vi "T7MOD_Write_with_Readback_UINT16_Register.vi"(6 "Timeout":u32=1000, 7 "UINT16 to Write":u16, 8 "error in":errorcluster, 9 "LabJack UINT16 Register":i32=55110, 10 "Remote Port":u16=502, 11 "Remote IP Address":string="192.168.1.15") -> (0 "error out":errorcluster, 1 "Written At":timestamp, 3 "nIter":i32)   [LabVIEW 2016]
panel:
  # "Input"
  # "TCP Parameters"
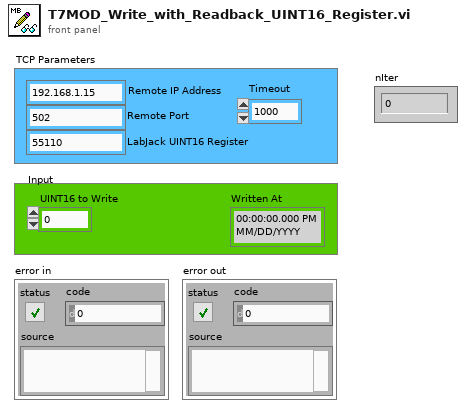
[diagram p1: front panel]
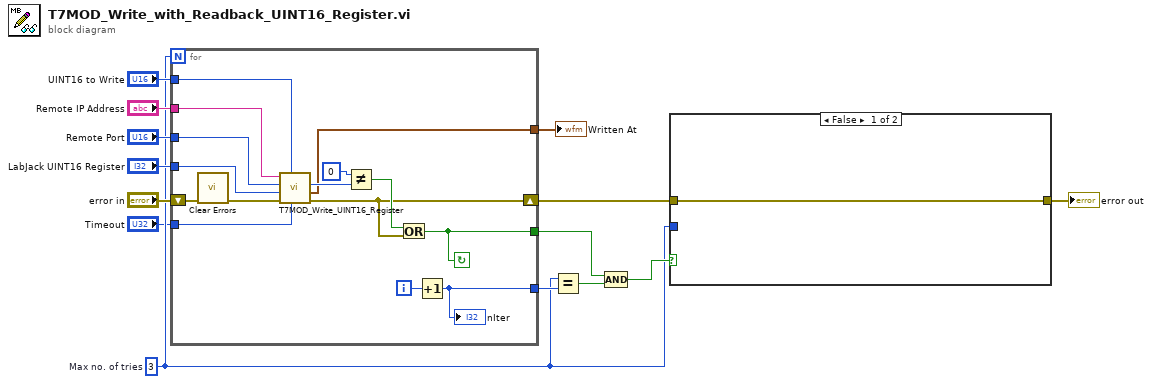
[diagram p0: block diagram]
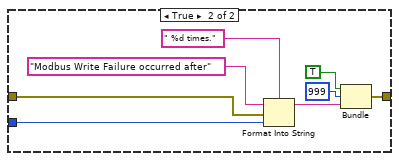
[diagram p2: hidden frame]
diagram:
  w6 = 3  # Max no. of tries
  n1 = for {
    N: w6 -> [_]
    tunnel: "Remote IP Address" -> [w29]
    shift-right: [w19] -> w4
    shift-left: "error in" -> [w16]
    tunnel: "Remote Port" -> [w28]
    tunnel: "LabJack UINT16 Register" -> [w27]
    tunnel: "UINT16 to Write" -> [w26]
    tunnel: [w23] -> w9
    tunnel: "Timeout" -> [w24]
    tunnel: [w18] -> w2
    tunnel: [w17] -> w1
    i -> [w25]
    stop <- w18 continue-if-true
    n2 = call <vilib>:"Clear Errors.vi"("error in (no error)"=w16) -> ("error out"=w15:errorcluster)  [unwired: 5 in, 1 out]
    n3 = call "T7MOD_Write_UINT16_Register.vi"("Timeout"=w24, "UINT16 to Write"=w26, "error in"=w15, "LabJack UINT16 Register"=w27, "Remote Port"=w28, "Remote IP Address"=w29) -> ("error out"=w19:errorcluster, "Written At"=w17:timestamp, "Exception Code"=w21:u8)  [unwired: 3 in]
    n4 = Not Equal?(x=u8 0 ("Exception Code"), y=w21) -> (x != y?=w20:bool)
    n5 = Or(x=w20, y=w19) -> (x .or. y?=w18:bool)
    n6 = Increment(x=w25) -> (x+1=w23:i32)
    "nIter" <- w23
  }
  "Written At" <- w1
  n7 = Equal?(x=w6, y=w9) -> (x = y?=w8:bool)
  n8 = Compound Arithmetic op=AND(w2, w8) -> (w7:bool)
  n9 = case shown="False" w7 {
    tunnel: w6 -> [_ w38]
    tunnel: w4 -> [w30 w35]
    tunnel: [w30 w31] -> w3
    frame False {
    }
    frame True {
      n10 = Format Into String(format string=" %d times.", initial string="Modbus Write Failure occurred after", error in=w35, w38) -> (resulting string=w32:string)  [unwired: 1 out]
      n11 = Bundle("status"=TRUE, "code"=999, w32) -> (w31:cluster{"status":bool, "code":i32, string})  [unwired: 1 in]
    }
  }
  "error out" <- w3
